vi "Get CITIPackage Info.vi"(8 "error in (no error)":errorcluster, 11 "CITI Package Refnum in":refnum<k24>) -> (0 "error out":errorcluster, 3 "CITI Package":T1)   [LabVIEW 2023, in "NI_HFNetworkAnalysis.lvlib"]
uses:
  NI_HFNetworkAnalysis.lvlib
  C:/srd-semi-rfcal-software/AuxTools/STSRFFixtureCharactUtility/Source/Code Modules/Fixture/Dependencies/HFNetworkAnalysis/Support Files/NACE.Utils.Data.dll
  Support Files/NACE.Utils.Data.dll
  Controls/CITI Package.ctl
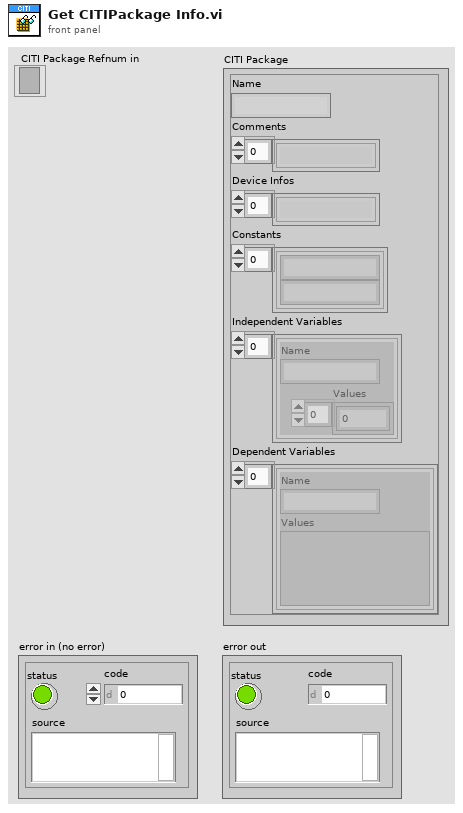
[diagram p1: front panel]
types:
  T1 = typedef "NI_HFNetworkAnalysis.lvlib/CITI Package.ctl" = cluster{"Name":string, "Comments":string[], "Device Infos":string[], "Constants":cluster{"Name":string, "Value":string}[], "Independent Variables":cluster{"Name":string, "Values":dbl[]}[], "Dependent Variables":cluster{"Name":string, "Values":variant}[]}
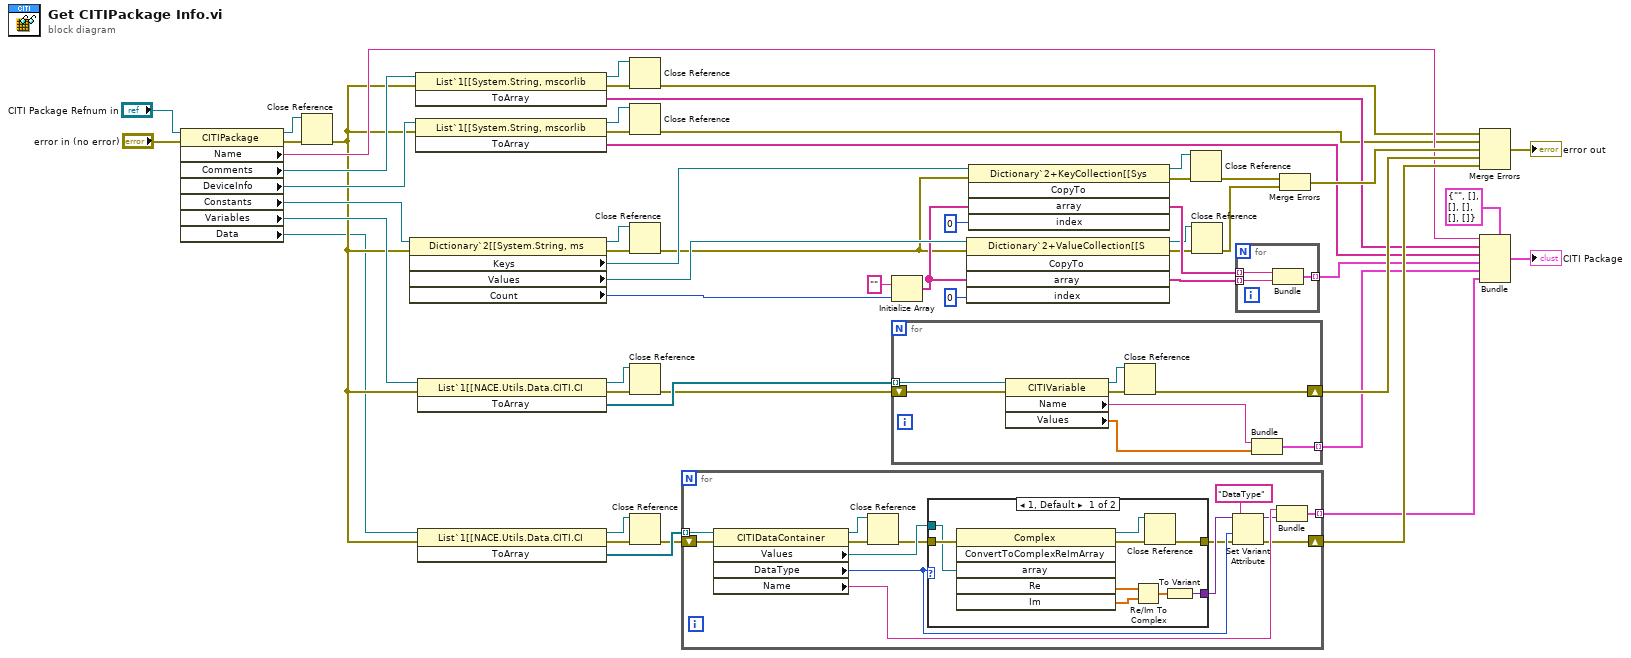
[diagram p0: block diagram]
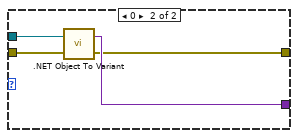
[diagram p2: hidden frame]
diagram:
  n1 = property class="CITIPackage"(reference="CITI Package Refnum in", error in="error in (no error)") -> (reference out=w4:refnum<k24>, error out=w54:errorcluster, "Name"=w26:string, "Comments"=w35:refnum<k24>, "DeviceInfo"=w34:refnum<k24>, "Constants"=w33:refnum<k24>, "Variables"=w32:refnum<k24>, "Data"=w2:refnum<k24>)
  n2 = Close Reference(reference=w4, error in (no error)=w54) -> (error out=w5:errorcluster)
  n3 = property class="Dictionary`2[[System.String, ms"(reference=w33, error in=w5) -> (reference out=w10:refnum<k24>, error out=w45:errorcluster, "Keys"=w47:refnum<k24>, "Values"=w44:refnum<k24>, "Count"=w40:i32)
  n4 = invoke class="List`1[[System.String, mscorlib" method="ToArray"(reference=w35, error in=w5) -> (reference out=w18:refnum<k24>, error out=w31:errorcluster, "ToArray"=w25:string[])  [unwired: 1 in]
  n5 = invoke class="List`1[[System.String, mscorlib" method="ToArray"(reference=w34, error in=w5) -> (reference out=w16:refnum<k24>, error out=w30:errorcluster, "ToArray"=w24:string[])  [unwired: 1 in]
  n6 = invoke class="List`1[[NACE.Utils.Data.CITI.CI" method="ToArray"(reference=w32, error in=w5) -> (reference out=w8:refnum<k24>, error out=w49:errorcluster, "ToArray"=w50:refnum<k24>[])  [unwired: 1 in]
  n7 = invoke class="List`1[[NACE.Utils.Data.CITI.CI" method="ToArray"(reference=w2, error in=w5) -> (reference out=w6:refnum<k24>, error out=w52:errorcluster, "ToArray"=w51:refnum<k24>[])  [unwired: 1 in]
  n8 = Close Reference(reference=w18, error in (no error)=w31) -> (error out=w19:errorcluster)
  n9 = Close Reference(reference=w16, error in (no error)=w30) -> (error out=w17:errorcluster)
  n10 = Close Reference(reference=w10, error in (no error)=w45) -> (error out=w11:errorcluster)
  n11 = Close Reference(reference=w8, error in (no error)=w49) -> (error out=w9:errorcluster)
  n12 = Close Reference(reference=w6, error in (no error)=w52) -> (error out=w7:errorcluster)
  n13 = for {
    tunnel: w51 -> [w66] mode=indexing
    tunnel: [w67] -> w21 mode=indexing
    shift-right: [w55] -> w27
    shift-left: w7 -> [w68]
    n14 = property class="CITIDataContainer"(reference=w66, error in=w68) -> (reference out=w61:refnum<k24>, error out=w63:errorcluster, "Values"=w64:refnum<k24>, "DataType"=w57:i32, "Name"=w65:string)
    n15 = Close Reference(reference=w61, error in (no error)=w63) -> (error out=w62:errorcluster)
    n16 = case shown="1, Default" w57 {
      tunnel: w64 -> [w76 w80]
      tunnel: w62 -> [w77 w81]
      tunnel: [w70 w78] -> w56
      tunnel: [w75 w79] -> w59
      frame 1, Default {
        n17 = invoke class="Complex" method="ConvertToComplexReImArray"(error in=w77, "array"=w76) -> (reference out=w69:refnum<k24>, error out=w74:errorcluster, "Re"=w73:dbl[], "Im"=w72:dbl[])  [unwired: 4 in, 2 out]
        n18 = Re/Im To Complex(1:w72, 2:w73) -> (0:w71:cdb[])
        n19 = Close Reference(reference=w69, error in (no error)=w74) -> (error out=w70:errorcluster)
        n20 = To Variant(anything=w71) -> (Variant=w75:variant)
      }
      frame 0 {
        n21 = call <vilib>:".NET Object To Variant.vi"("error in (no error)"=w81, ".NET object"=w80) -> ("error out"=w78:errorcluster, "variant"=w79:variant)
      }
    }
    n22 = Set Variant Attribute(Variant=w59, name="DataType", value=w57, error in=w56) -> (Variant out=w58:variant, error out=w55:errorcluster)  [unwired: 1 out]
    n23 = Bundle("Name"=w65, "variant"=w58) -> (w67:cluster{"Name":string, "variant":variant})  [unwired: 1 in]
  }
  n24 = Initialize Array("", w40) -> (w38:string[])
  n25 = for {
    tunnel: w50 -> [w88] mode=indexing
    tunnel: [w89] -> w22 mode=indexing
    shift-right: [w83] -> w28
    shift-left: w9 -> [w87]
    n26 = property class="CITIVariable"(reference=w88, error in=w87) -> (reference out=w82:refnum<k24>, error out=w86:errorcluster, "Name"=w85:string, "Values"=w84:dbl[])
    n27 = Close Reference(reference=w82, error in (no error)=w86) -> (error out=w83:errorcluster)
    n28 = Bundle("Name"=w85, "Values"=w84) -> (w89:cluster{"Name":string, "Values":dbl[]})  [unwired: 1 in]
  }
  n29 = invoke class="Dictionary`2+ValueCollection[[S" method="CopyTo"(reference=w44, error in=w11, "array"=w38, "index"=0) -> (reference out=w12:refnum<k24>, error out=w36:errorcluster, "array"=w41:string[])  [unwired: 1 in, 2 out]
  n30 = invoke class="Dictionary`2+KeyCollection[[Sys" method="CopyTo"(reference=w47, error in=w11, "array"=w38, "index"=0) -> (reference out=w14:refnum<k24>, error out=w37:errorcluster, "array"=w42:string[])  [unwired: 1 in, 2 out]
  n31 = Close Reference(reference=w14, error in (no error)=w37) -> (error out=w15:errorcluster)
  n32 = Close Reference(reference=w12, error in (no error)=w36) -> (error out=w13:errorcluster)
  n33 = for {
    tunnel: [w92] -> w23 mode=indexing
    tunnel: w42 -> [w91] mode=indexing
    tunnel: w41 -> [w90] mode=indexing
    n34 = Bundle(w91, w90) -> (w92:cluster{string, string})  [unwired: 1 in]
  }
  n35 = Merge Errors(w15, w13) -> (w29:errorcluster)
  n36 = Merge Errors(w19, w17, w29, w28, w27) -> (→"error out":errorcluster)
  n37 = Bundle(cluster=T1 {"Name"="", "Comments"=[], "Device Infos"=[], "Constants"=[], "Independent Variables"=[], "Dependent Variables"=[]} ("CITI Package"), "Name"=w26, "Comments"=w25, "Device Infos"=w24, "Constants"=w23, "Independent Variables"=w22, "Dependent Variables"=w21) -> (→"CITI Package":T1)
